vi "RT Combined SAR and DSA.vi"() -> ()   [LabVIEW 2025]
uses:
  <vilib>/FPGAPlugInAG/cRIO-9045/niLvFpga_Open_cRIO-9045.vi
  <vilib>/rvi/interface/common/dynamic/niFpgaDynamicAddResources.vi
  <vilib>/rvi/interface/common/niFpgaWaitOnOcc.vi
  <vilib>/Utility/error.llb/Error Cluster From Error Code.vi
  <vilib>/FPGAPlugInAG/Dynamic/niLvFpga_Run_Dynamic.vi
  <vilib>/rvi/errors/niLvFpgaAdjustHostInterfaceError.vi
  <vilib>/FPGAPlugInAG/Dynamic/niLvFpga_Close_Dynamic.vi
  <vilib>/rvi/interface/nirviOpenFPGA/nirviOpenFPGA.xnode
  FPGA Bitfiles/basicioaccess_FPGATarget_FPGACombinedSARa_+zXWa+NKGwk.lvbitx
  <vilib>/rvi/interface/nirviMethod/nirviMethod.xnode
  <vilib>/rvi/interface/nirviReadWriteControl/nirviReadWriteControl.xnode
  <vilib>/rvi/interface/nirviCloseFPGA/nirviCloseFPGA.xnode
  <vilib>/FPGAPlugInAG/Dynamic/niLvFpga_ConfigureFifo_Dynamic.vi
  <vilib>/rvi/errors/niLvFpgaMergeErrorWithErrorCode.vi
  <vilib>/FPGAPlugInAG/Dynamic/niLvFpga_StartFifo_Dynamic.vi
  NiFpgaLv.dll
  <vilib>/rvi/interface/Simulation/niFpgaSimulationCallBeginRW.vi
  <vilib>/FPGAPlugInAG/Dynamic/niLvFpga_ReadFifo_Dynamic.vi
  <vilib>/FPGAPlugInAG/Dynamic/niLvFpga_StopFifo_Dynamic.vi
panel:
  out "error out":errorcluster
  in  "stop DMA":bool
  out "Waveform Graph":sgl[][](graph)
  in  "stop read / write":bool
  out "Mod2/DIO0":bool
  out "Mod2/DIO1":bool
  out "Mod2/DIO2":bool
  out "Mod2/DIO3":bool
  in  "Mod1/DO0":bool
  in  "Mod1/DO1":bool
  in  "Mod1/DO2":bool
  in  "Mod1/DO3":bool
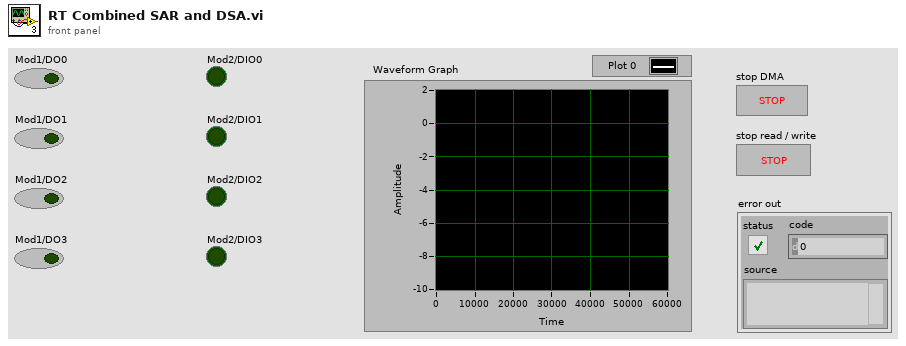
[diagram p1: front panel]
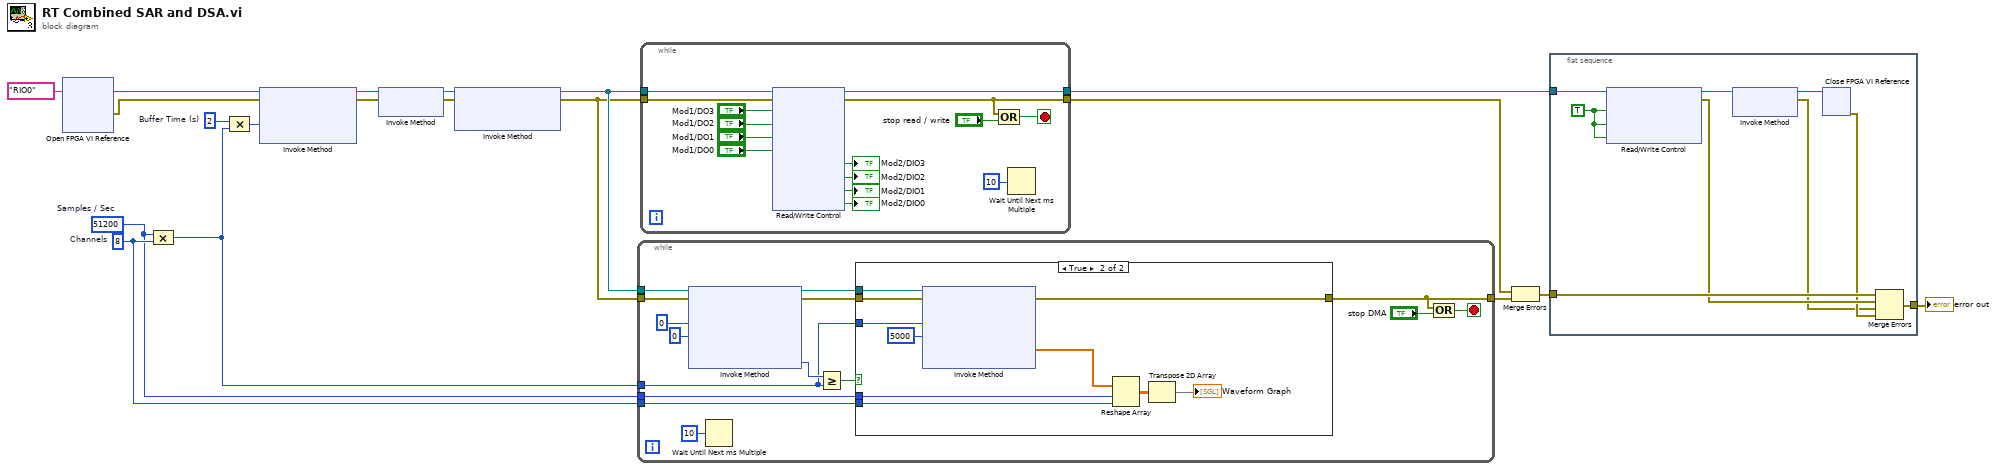
[diagram p0: block diagram]
diagram:
  w9 = u32 2  # Buffer Time (s)
  w6 = u32 8  # Channels
  w5 = u32 51200  # Samples / Sec
  n1 = xnode "Open FPGA VI Reference"("resource name"=tag "RIO0") -> ("FPGA VI Reference Out"=w18:refnum<k20>, "error out"=w17:errorcluster)  [unwired: 1 in]
  n2 = Compound Arithmetic op=MULTIPLY(w5, w6) -> (w7:u32)
  n3 = Compound Arithmetic op=MULTIPLY(w9, w7) -> (w8:u32)
  n4 = xnode "Invoke Method"("FPGA VI Reference In"=w18, "error in"=w17, "Requested Depth"=w8) -> ("FPGA VI Reference Out"=w16:refnum<k20>, "error out"=w15:errorcluster)  [unwired: 1 out]
  n5 = xnode "Invoke Method"("FPGA VI Reference In"=w16, "error in"=w15) -> ("FPGA VI Reference Out"=w14:refnum<k20>, "error out"=w13:errorcluster)
  n6 = xnode "Invoke Method"("FPGA VI Reference In"=w14, "error in"=w13) -> ("FPGA VI Reference Out"=w11:refnum<k20>, "error out"=w10:errorcluster)  [unwired: 1 in]
  n7 = while {
    tunnel: w11 -> [w34]
    tunnel: w10 -> [w33]
    tunnel: w7 -> [w26]
    tunnel: w6 -> [w25]
    tunnel: w5 -> [w24]
    tunnel: [w20] -> w3
    stop <- w21 stop-if-true
    n8 = xnode "Invoke Method"("FPGA VI Reference In"=w34, "error in"=w33, "Number of Elements"=u32 0, "Timeout (ms)"=0) -> ("FPGA VI Reference Out"=w28:refnum<k20>, "error out"=w27:errorcluster, "Elements Remaining"=w31:u32)  [unwired: 1 out]
    n9 = Wait Until Next ms Multiple(millisecond multiple=u32 10) -> ()  [unwired: 1 out]
    n10 = Greater Or Equal?(x=w31, y=w26) -> (x >= y?=w30:bool)
    n11 = case shown="True" w30 {
      tunnel: w28 -> [_ w45]
      tunnel: w27 -> [w35 w44]
      tunnel: w26 -> [_ w43]
      tunnel: w25 -> [_ w39]
      tunnel: w24 -> [_ w38]
      tunnel: [w35 w36] -> w20
      frame False {
      }
      frame True {
        n12 = xnode "Invoke Method"("FPGA VI Reference In"=w45, "error in"=w44, "Number of Elements"=w43, "Timeout (ms)"=5000) -> ("error out"=w36:errorcluster, "Data"=w40:sgl[])  [unwired: 2 out]
        n13 = Reshape Array(w40, w38, w39) -> (w41:sgl[][])
        n14 = Transpose 2D Array(2D array=w41) -> (transposed array=→"Waveform Graph":sgl[][])
      }
    }
    n15 = Compound Arithmetic op=OR(w20, "stop DMA") -> (w21:bool)
  }
  n16 = while {
    tunnel: w11 -> [w60]
    tunnel: w10 -> [w59]
    tunnel: [w48] -> w12
    tunnel: [w46] -> w4
    stop <- w49 stop-if-true
    n17 = xnode "Read/Write Control"("FPGA VI Reference In"=w60, "error in"=w59, "Mod1/DO3"="Mod1/DO3", "Mod1/DO2"="Mod1/DO2", "Mod1/DO1"="Mod1/DO1", "Mod1/DO0"="Mod1/DO0") -> ("FPGA VI Reference Out"=w48:refnum<k20>, "error out"=w46:errorcluster, "Mod2/DIO3"=→"Mod2/DIO3":bool, "Mod2/DIO2"=→"Mod2/DIO2":bool, "Mod2/DIO1"=→"Mod2/DIO1":bool, "Mod2/DIO0"=→"Mod2/DIO0":bool)
    n18 = Compound Arithmetic op=OR(w46, "stop read / write") -> (w49:bool)
    n19 = Wait Until Next ms Multiple(millisecond multiple=u32 10) -> ()  [unwired: 1 out]
  }
  n20 = Merge Errors(w4, w3) -> (w2:errorcluster)
  n21 = flat-sequence {
    tunnel: w12 -> [w69]
    tunnel: w2 -> [w67]
    tunnel: [w65] -> w1
    frame #0 {
      w68 = TRUE ("stop Slow Digital")
      n22 = xnode "Read/Write Control"("FPGA VI Reference In"=w69, "stop Slow Digital"=w68, "stop Combined"=w68, "stop Fast Digital"=w68) -> ("FPGA VI Reference Out"=w64:refnum<k20>, "error out"=w66:errorcluster)  [unwired: 1 in]
      n23 = xnode "Invoke Method"("FPGA VI Reference In"=w64) -> ("FPGA VI Reference Out"=w63:refnum<k20>, "error out"=w61:errorcluster)  [unwired: 1 in]
      n24 = xnode "Close FPGA VI Reference"("FPGA VI Reference In"=w63) -> ("error out"=w62:errorcluster)  [unwired: 1 in]
      n25 = Merge Errors(w67, w66, w61, w62) -> (w65:errorcluster)
    }
  }
  "error out" <- w1
